vi "uc480_SetFramerate.vi"(0 ".NET (Reference)":refnum<k24>, 7 "Frame rate":dbl, 11 "Error In":errorcluster) -> (15 "Error out":errorcluster caption="Error Out")   [LabVIEW 2021]
uses:
  C:/Program Files/Thorlabs/Scientific Imaging/ThorCam/uc480DotNet.dll
  Program Files/Thorlabs/Scientific Imaging/ThorCam/uc480DotNet.dll
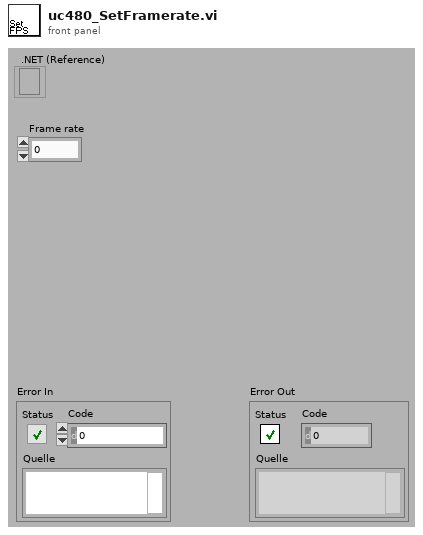
[diagram p1: front panel]
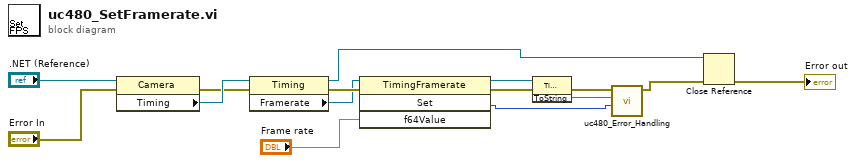
[diagram p0: block diagram]
diagram:
  n1 = property class="Camera"(reference=".NET (Reference)", error in="Error In") -> (error out=w14:errorcluster, "Timing"=w15:refnum<k24>)  [unwired: 1 out]
  n2 = property class="Timing"(reference=w15, error in=w14) -> (reference out=w8:refnum<k24>, error out=w13:errorcluster, "Framerate"=w12:refnum<k24>)
  n3 = invoke class="TimingFramerate" method="Set"(reference=w12, error in=w13, "f64Value"="Frame rate") -> (reference out=w6:refnum<k24>, error out=w5:errorcluster, "Set"=w2:i32)  [unwired: 1 in, 1 out]
  n4 = invoke class="TimingFramerate" method="ToString"(reference=w6, error in=w5) -> (error out=w4:errorcluster, "ToString"=w3:string)  [unwired: 1 in, 1 out]
  n5 = call "uc480_Error_Handling.vi"("Error Code"=w2, "Error String"=w3, "Error In"=w4) -> ("Error Out"=w1:errorcluster)  [unwired: 8 in]
  n6 = Close Reference(reference=w8, error in (no error)=w1) -> (error out=→"Error out":errorcluster)
